vi "PID_TempControl_GCFS.vi"(5 "CheckResponse?":bool, 6 "reinitialize? (F)":bool, 7 "Manual Temp Control.Active":bool, 10 "Temperature":dbl, 11 "?":T1={"Core"={"Current VI Reference"=refnum, "Close Panel on Exit?"=FALSE}, "Your Boolean data"=FALSE, "Your string data"="", "Camera Cluster"={"Session"="", "Image"=refnum, "Position Image"=refnum, "PixelVal Image"=refnum, "Position Image Binary"=refnum, "Lable Image"=refnum, "Merged Image"=refnum, "Connection"=FALSE}, "Data In Cluster"={"Images"={"Position Image path"=path "", "Sample folder path"=path "", "Label Image path"=path ""}, "Sample Name"="", "Sample Rate"=0, "Gradient Buffer"=0, "Data Acquisition.Setup.TempGrad"=0.0, "Control.PID gains"={"proportional gain (Kc)"=0.0, "integral time (Ti, min)"=0.0, "derivative time (Td, min)"=0.0}, "Freezing value"=250.0}, "Active"=FALSE, "Ready"=FALSE, "Exit"=FALSE, "Arduino"={"Connection"=FALSE, "Port"="", "State"=""}, "Program_Start"="", "Data Out Cluster"={"Particle Measurements"=[], "Number of droplets"=0, "PosImg_Timestamp"="", "OverlayProp"=[], "Group"="", "Que"=refnum}, "PSU"={"Connection"=FALSE, "Port"="", "State"=""}, "Load Rerun"=FALSE, "Rerun"=FALSE, "cDAQ"={"Connection"=FALSE, "ID"="", "Task"=""}} {"Data Out Cluster"."Particle Measurements" format="%.2f"}) -> (0 "error out":errorcluster, 1 "valid?":bool, 2 "Temp Gradient":dbl, 3 "Output%":dbl format="%.2f")   [LabVIEW 2024]
uses:
  Micro/DataCluster_GCFS.ctl
  <vilib>/userDefined/High Color/IMAQdx.ctl
  <vilib>/vision/Image Controls.llb/IMAQ Image.ctl
  <vilib>/vision/Image Controls.llb/Overlay Property.ctl
  ee7b73c5-abbe-409c-97f6-86d988c3f229.vi
  <vilib>/addons/control/pid/pid.llb/PID (DBL).vi
  <vilib>/regexp/Match Regular Expression.xnode
  <vilib>/addons/control/pid/NI_PID_pid.lvlib
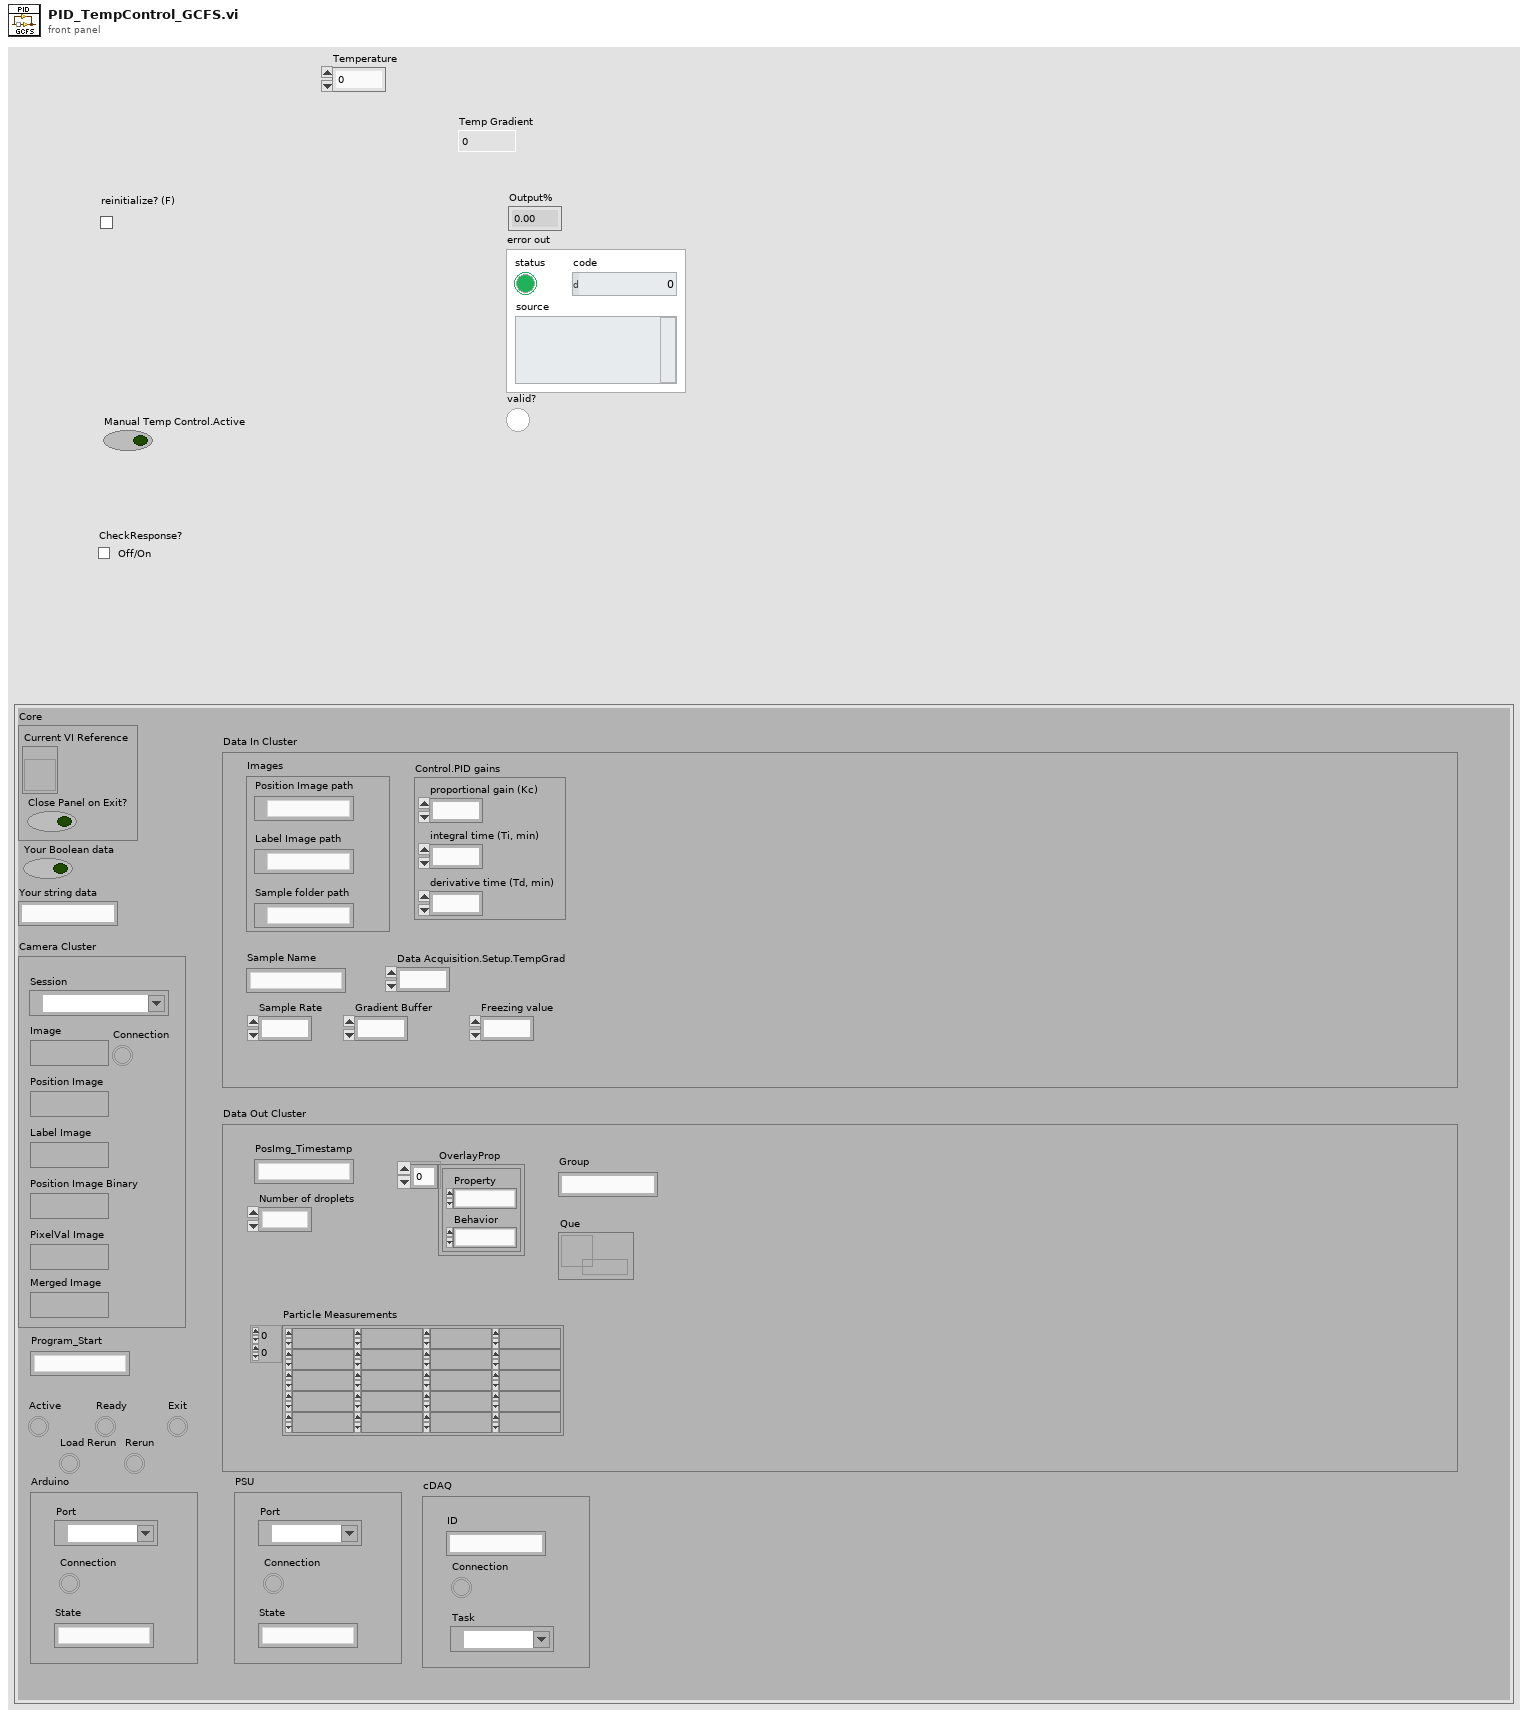
[diagram p1: front panel]
types:
  T1 = typedef "DataCluster_GCFS.ctl" = cluster{"Core":cluster{"Current VI Reference":refnum<vi>, "Close Panel on Exit?":bool}, "Your Boolean data":bool, "Your string data":string, "Camera Cluster":cluster{"Session":T2, "Image":T3, "Position Image":T3, "PixelVal Image":T3, "Position Image Binary":T3, "Lable Image":T3, "Merged Image":T3, "Connection":bool}, "Data In Cluster":cluster{"Images":cluster{"Position Image path":path, "Sample folder path":path, "Label Image path":path}, "Sample Name":string, "Sample Rate":i32, "Gradient Buffer":i32, "Data Acquisition.Setup.TempGrad":dbl, "Control.PID gains":cluster{"proportional gain (Kc)":dbl, "integral time (Ti, min)":dbl, "derivative time (Td, min)":dbl}, "Freezing value":sgl}, "Active":bool, "Ready":bool, "Exit":bool, "Arduino":cluster{"Connection":bool, "Port":refnum<visa-resource-name>, "State":string}, "Program_Start":string, "Data Out Cluster":cluster{"Particle Measurements":dbl[][], "Number of droplets":i32, "PosImg_Timestamp":string, "OverlayProp":T4[], "Group":string, "Que":refnum<queue>}, "PSU":cluster{"Connection":bool, "Port":refnum<visa-resource-name>, "State":string}, "Load Rerun":bool, "Rerun":bool, "cDAQ":cluster{"Connection":bool, "ID":string, "Task":refnum<k21>}}
  T2 = typedef "IMAQdx.ctl" = refnum<k21>
  T3 = typedef "IMAQ Image.ctl" = refnum<image>
  T4 = typedef "Overlay Property.ctl" = cluster{"Property":enum32{"Scale", "Shift", "Rotate", "Symmetry"}, "Behavior":enum32{"Clear", "Keep", "Transform"}}
  T5 = cluster{"proportional gain (Kc)":dbl, "integral time (Ti, min)":dbl, "derivative time (Td, min)":dbl}
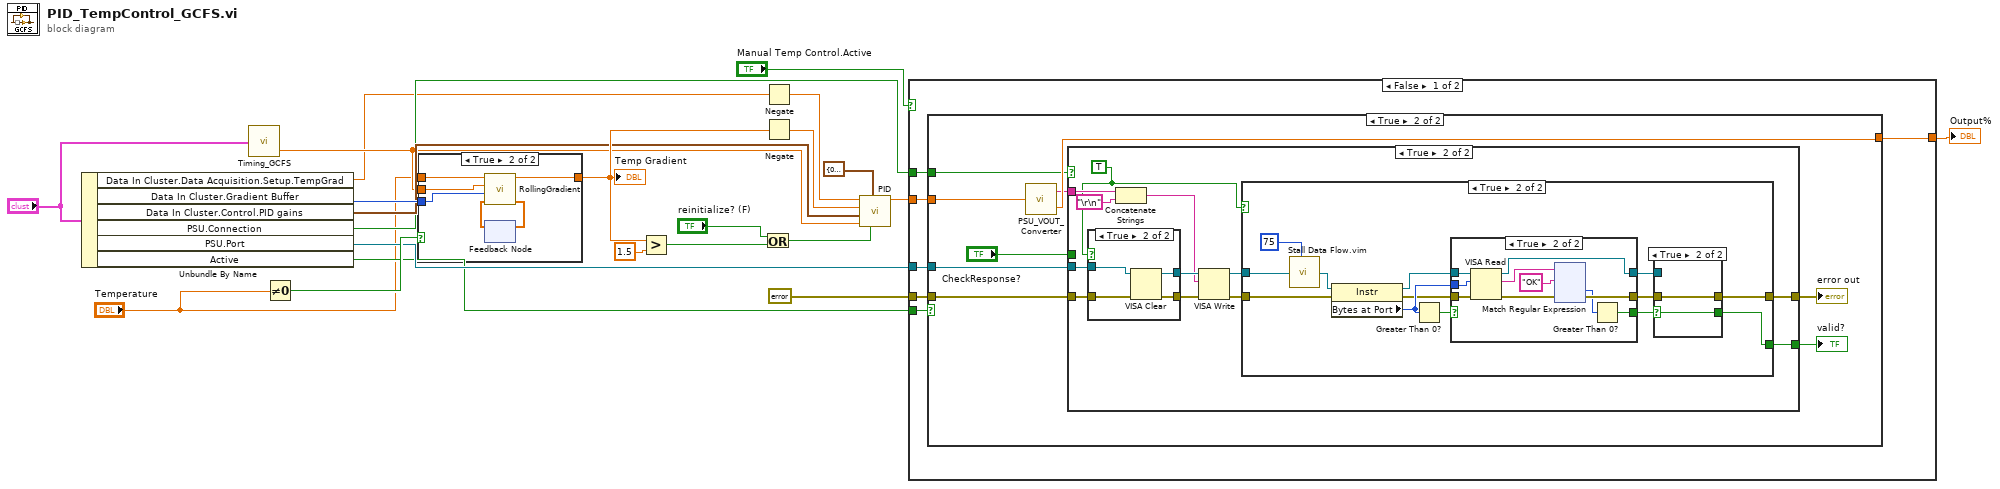
[diagram p0: block diagram]
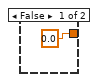
[diagram p2: hidden frame]
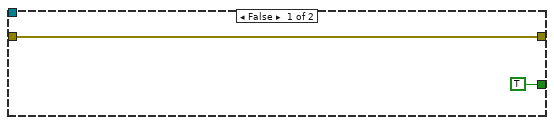
[diagram p5: hidden frame]
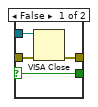
[diagram p6: hidden frame]
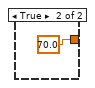
[diagram p8: hidden frame]
diagram:
  n1 = Unbundle By Name("?") -> ("Data In Cluster.Data Acquisition.Setup.TempGrad"=w2:dbl, "Data In Cluster.Gradient Buffer"=w11:i32, "Data In Cluster.Control.PID gains"=w10:T5, "PSU.Connection"=w9:bool, "PSU.Port"=w8:refnum<visa-resource-name>, "Active"=w7:bool)
  n2 = call "Timing_GCFS.vi"(0:"?") -> ("Sample dt (s)"=w5:dbl)  [unwired: 1 out]
  n3 = Not Equal To 0?(x="Temperature") -> (x != 0?=w22:bool)
  n4 = case shown="True" w22 {
    tunnel: w5 -> [_ w27]
    tunnel: [_ w26] -> w14
    tunnel: "Temperature" -> [_ w28]
    tunnel: w11 -> [_ w25]
    frame False {
    }
    frame True {
      n5 = feedback #1() -> (w24:dbl[])  [unwired: 1 in]
      n6 = call "RollingGradient.vi"("TempArray in"=w24, "FitSize"=w25, "dt"=w27, "mean temp"=w28) -> ("TempArray"=w23:dbl[], "gradient"=w26:dbl)  [unwired: 6 in]
      n7 = feedback-in #1(w23) -> ()
    }
  }
  "Temp Gradient" <- w14
  n8 = Greater?(x=w14, y=1.5) -> (0:w20:bool)
  n9 = Or(x="reinitialize? (F)", y=w20) -> (x .or. y?=w13:bool)
  n10 = Negate(x=w2) -> (-x=w17:dbl)
  n11 = Negate(x=w14) -> (-x=w15:dbl)
  n12 = call-poly <vilib>:"PID.vi"("reinitialize? (F)"=w13, "output range"=cluster{"output high":dbl, "output low":dbl} {"output high"=0.0, "output low"=100.0}, "dt (s)"=w5, "PID gains"=w10, "process variable"=w15, "setpoint"=w17) -> ("output"=w4:dbl)  [unwired: 4 in, 1 out]
  n13 = case shown="False" "Manual Temp Control.Active" {
    tunnel: w4 -> [w34 _]
    tunnel: [w33 70.0 ("Output % duplicate")] -> w18
    tunnel: w7 -> [w32 _]
    tunnel: w9 -> [w31 _]
    tunnel: w8 -> [w30 _]
    tunnel: errorcluster {"status"=FALSE, "code"=0, "source"=""} ("error in (no error)") -> [w29 _]
    frame False {
      n14 = case shown="True" w32 {
        tunnel: w34 -> [_ w41]
        tunnel: [0.0 ("Output % duplicate") w40] -> w33
        tunnel: w31 -> [_ w39]
        tunnel: w30 -> [_ w38]
        tunnel: w29 -> [_ w36]
        frame False {
        }
        frame True {
          n15 = call "PSU_VOUT_Converter.vi"("Output %"=w41) -> ("decimal integer string"=w37:string, "Output % duplicate"=w40:dbl)
          n16 = case shown="True" w39 {
            selector: w39 -> [w46 _]
            tunnel: w38 -> [_ w57]
            tunnel: [w45 w51] -> w44
            tunnel: [w46 w50] -> w43
            tunnel: w37 -> [_ w52]
            tunnel: "CheckResponse?" -> [_ _]
            tunnel: w36 -> [w45 w48]
            frame False {
            }
            frame True {
              w47 = TRUE
              n17 = case shown="True" w47 {
                tunnel: w57 -> [w60 w64]
                tunnel: [w60 w63] -> w56
                tunnel: [w59 w62] -> w55
                tunnel: w48 -> [w59 w61]
                frame False {
                }
                frame True {
                  n18 = VISA Clear(VISA resource name=w64, error in (no error)=w61) -> (VISA resource name out=w63:refnum<visa-resource-name>, error out=w62:errorcluster)
                }
              }
              n19 = Concatenate Strings(w52, "\r\n") -> (w49:string)
              n20 = VISA Write(VISA resource name=w56, write buffer=w49, error in (no error)=w55) -> (VISA resource name out=w54:refnum<visa-resource-name>, error out=w53:errorcluster)  [unwired: 1 out]
              n21 = case shown="True" w47 {
                tunnel: w54 -> [_ w73]
                tunnel: w53 -> [w65 w72]
                tunnel: [w65 w70] -> w51
                tunnel: [TRUE w68] -> w50
                frame False {
                }
                frame True {
                  n22 = call "Stall Data Flow.vim"("value in"=w73, "milliseconds to wait"=u32 75) -> ("value out"=w79:refnum<visa-resource-name>)  [unwired: 1 out]
                  n23 = property class="Instr"(reference=w79, error in=w72) -> (reference out=w76:refnum<visa-resource-name>, error out=w75:errorcluster, "Bytes at Port"=w77:u32)
                  n24 = Greater Than 0?(x=w77) -> (x > 0?=w78:bool)
                  n25 = case shown="True" w78 {
                    selector: w78 -> [w87 _]
                    tunnel: w77 -> [_ w98]
                    tunnel: w75 -> [w88 w97]
                    tunnel: [w88 w92] -> w69
                    tunnel: w76 -> [w86 w96]
                    tunnel: [w87 w90] -> w71
                    tunnel: [w86 w89] -> w67
                    frame False {
                    }
                    frame True {
                      n26 = VISA Read(VISA resource name=w96, byte count=w98, error in (no error)=w97) -> (VISA resource name out=w89:refnum<visa-resource-name>, read buffer=w95:string, error out=w94:errorcluster)  [unwired: 1 out]
                      n27 = xnode "Match Regular Expression"("input string"=w95, "regular expression"="OK", "error in"=w94) -> ("offset past match"=w91:i32, "error out"=w92:errorcluster)  [unwired: 3 in, 3 out]
                      n28 = Greater Than 0?(x=w91) -> (x > 0?=w90:bool)
                    }
                  }
                  n29 = case shown="True" w71 {
                    selector: w71 -> [w83 w84]
                    tunnel: [w80 w85] -> w70
                    tunnel: w69 -> [w81 w85]
                    tunnel: [w83 w84] -> w68
                    tunnel: w67 -> [w82 _]
                    frame False {
                      n30 = VISA Close(VISA resource name=w82, error in (no error)=w81) -> (error out=w80:errorcluster)
                    }
                    frame True {
                    }
                  }
                }
              }
            }
          }
          "error out" <- w44
          "valid?" <- w43
        }
      }
    }
    frame True {
    }
  }
  "Output%" <- w18
